vi "_PC_Pub_Display_MSSignalInTime.vi"() -> (10 "System Waveform Chart":waveform(dbl)[](graph))   [LabVIEW 2016]
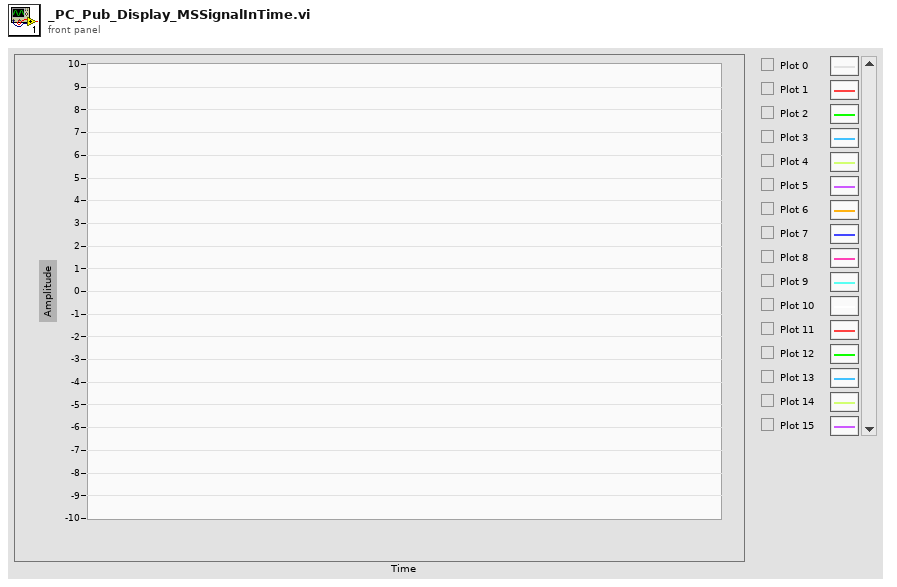
[diagram p1: front panel]
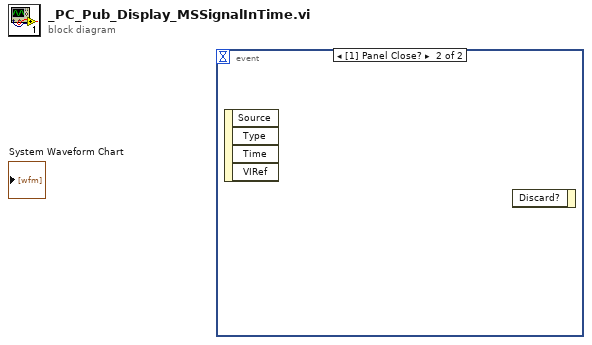
[diagram p0: block diagram]
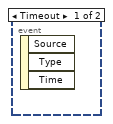
[diagram p2: hidden frame]
diagram:
  n1 = event shown="[1] Panel Close?" {
    selector: _ -> [_ _]
    dyn-events: _ -> [_ _]
    timeout: _ -> [_ _]
    event Timeout {
      n2 = event-data() -> ()  [unwired: 1 in, 3 out]
    }
    event Panel Close? {
      n3 = event-data() -> ()  [unwired: 1 in, 4 out]
      n4 = event-data() -> ()  [unwired: 2 in, 1 out]
    }
  }
